vi "json Parse Float - array path.vi"(8 "error in (no error)":errorcluster, 9 "default":sgl, 10 "path":string[](array[string]), 11 "JSON Document in":refnum<class "JSON Document.lvclass">) -> (0 "error out":errorcluster, 2 "value":sgl, 3 "JSON Document out":refnum<class "JSON Document.lvclass">)   [LabVIEW 2015, in "JSON Document.lvclass"]
uses:
  JSON Document.lvclass
  json Parse Float - string path.vi
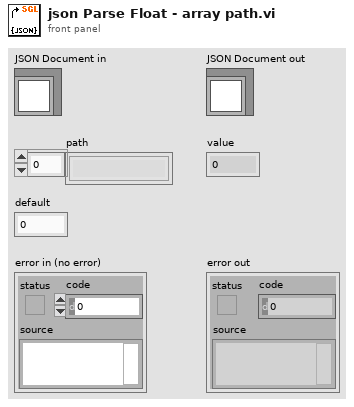
[diagram p1: front panel]
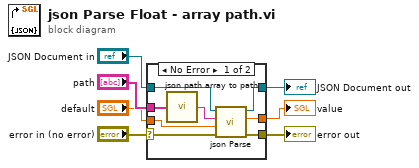
[diagram p0: block diagram]
diagram:
  n1 = case shown="No Error" "error in (no error)" {
    selector: "error in (no error)" -> [w8 w18]
    tunnel: [w9 w18] -> w3
    tunnel: [w11 w17] -> w1
    tunnel: "JSON Document in" -> [w15 w17]
    tunnel: "default" -> [w12 w16]
    tunnel: "path" -> [w14 _]
    tunnel: [w10 w16] -> w2
    frame No Error {
      n2 = call "json path array to path.vi"("path"=w14) -> ("String"=w13:string)
      n3 = call-poly "json Parse.vi"("error in (no error)"=w8, "default"=w12, "path"=w13, "JSON Document in"=w15) -> ("error out"=w9:errorcluster, "value"=w10:sgl, "JSON Document out"=w11:refnum<class "JSON Document.lvclass">)  [unwired: 5 in]
    }
    frame Error {
    }
  }
  "error out" <- w3
  "JSON Document out" <- w1
  "value" <- w2
